vi "MOTOR Configure Acceleration.vi"(8 "error in (no error)":errorcluster, 10 "Message Data":variant, 11 "Data Cluster in":T1={"Tango HW"={"VISA resource"="", "Baud Rate (115200)"=2, "lAnInterfaceType"=0, "bAShowProt"=15}, "Writer Queue"=refnum, "Status"=FALSE, "Abs Position"=[], "Axis Velocity"={"dX"=0.0, "dY"=0.0, "dZ"=0.0, "dA"=0.0}, "acceleration "=0.0, "Z direction"=enum."Up", "Position Mode"="", "plLSID"=0}) -> (0 "error out":errorcluster, 3 "Data Cluster out":T1={"Tango HW"={"VISA resource"="", "Baud Rate (115200)"=2, "lAnInterfaceType"=0, "bAShowProt"=15}, "Writer Queue"=refnum, "Status"=FALSE, "Abs Position"=[], "Axis Velocity"={"dX"=0.0, "dY"=0.0, "dZ"=0.0, "dA"=0.0}, "acceleration "=0.0, "Z direction"=enum."Up", "Position Mode"="", "plLSID"=0})   [LabVIEW 2020, in "MOTOR.lvlib"]
uses:
  MOTOR.lvlib
  PS Hardware Configuration.ctl
  support/Message Queue/Message Cluster.ctl
  support/HW Message Cluster.ctl
  support/PCT FGV CMD.ctl
  support/Message Queue/Message Queue.lvlib
  <instrlib>/Tango_DLL/Tango_DLL.lvlib
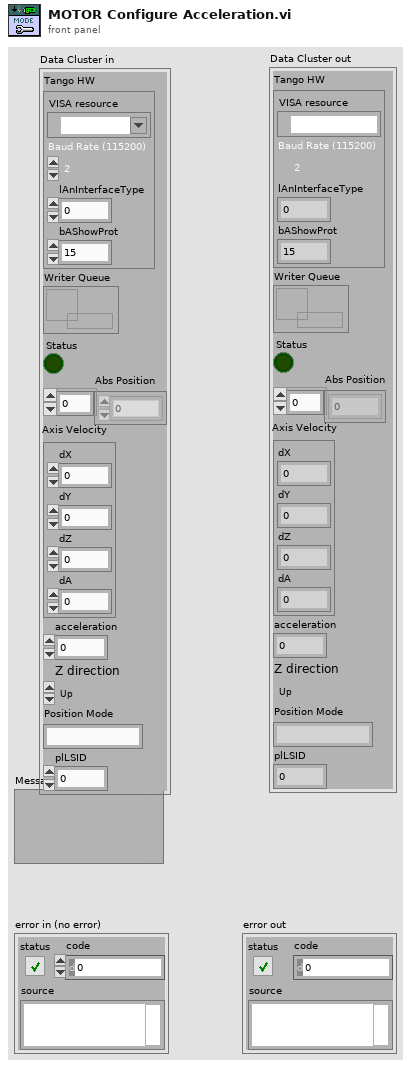
[diagram p1: front panel]
types:
  T1 = typedef "MOTOR.lvlib/PS Hardware Configuration.ctl" = cluster{"Tango HW":cluster{"VISA resource":refnum<visa-resource-name>, "Baud Rate (115200)":i32, "lAnInterfaceType":i32, "bAShowProt":i32}, "Writer Queue":refnum<queue>, "Status":bool, "Abs Position":i32[], "Axis Velocity":cluster{"dX":dbl, "dY":dbl, "dZ":dbl, "dA":dbl}, "acceleration ":dbl, "Z direction":enum16{"Up", "Down"}, "Position Mode":string, "plLSID":i32}
  T2 = typedef "PCT FGV CMD.ctl" = enum16{"INIT", "GET", "SET"}
  T3 = typedef "Message Queue.lvlib/HW Message Cluster.ctl" = cluster{"Writer Queue":refnum<queue>, "Writer Data":T4}
  T4 = typedef "Message Queue.lvlib/Message Cluster.ctl" = cluster{"Message":string, "Message Data":variant}
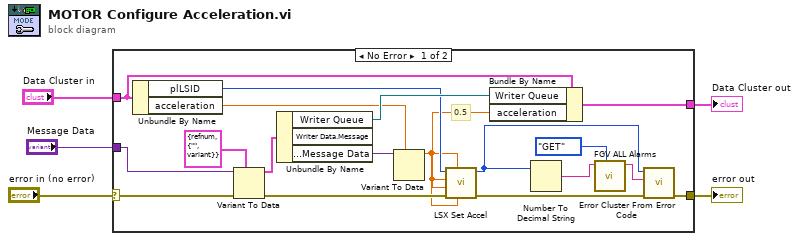
[diagram p0: block diagram]
diagram:
  n1 = case shown="No Error" "error in (no error)" {
    selector: "error in (no error)" -> [w20 w24]
    tunnel: "Message Data" -> [w19 _]
    tunnel: [w18 w25] -> w4
    tunnel: "Data Cluster in" -> [w16 w25]
    tunnel: [w12 w24] -> w2
    frame No Error {
      # "0.5"
      n2 = Unbundle By Name(w16) -> ("plLSID"=w10:i32, "acceleration"=w15:dbl)
      n3 = Variant To Data(error in=w20, type=T3 {"Writer Queue"=refnum, "Writer Data"={"Message"="", "Message Data"=variant}}, Variant=w19) -> (data=w23:T3, error out=w9:errorcluster)
      n4 = Unbundle By Name(w23) -> ("Writer Queue"=w22:refnum<queue>, "Writer Data.Message Data"=w17:variant)  [unwired: 1 out]
      n5 = Variant To Data(type=w15, Variant=w17) -> (data=w6:dbl)  [unwired: 1 in, 1 out]
      n6 = call <instrlib>:"LSX Set Accel.vi"("dA"=w6, "dZ"=w6, "error in (no error)"=w9, "dY"=w6, "dX"=w6, "lLSID"=w10) -> ("error out"=w7:errorcluster, "function return"=w8:i32)  [unwired: 4 in]
      n7 = Bundle By Name(cluster=w16, "Writer Queue"=w22, "acceleration"=w6) -> (w18:T1)
      n8 = Number To Decimal String(number=w8) -> (decimal integer string=w13:string)  [unwired: 1 in]
      n9 = call "FGV ALL Alarms.vi"("CMD"=PCT_FGV_CMD."GET", "name"=w13) -> ("Alarm MSG out"=w11:string)  [unwired: 8 in, 1 out]
      n10 = call <vilib>:"Error Cluster From Error Code.vi"("error in (no error)"=w7, "error message (\"\")"=w11, "error code (0)"=w8) -> ("error out"=w12:errorcluster)  [unwired: 6 in]
    }
    frame Error {
    }
  }
  "Data Cluster out" <- w4
  "error out" <- w2
